vi "EOM.vi"(8 "error in (no error)":errorcluster, 9 "USE EOM?":bool, 10 "EOM_amplitude":dbl, 11 "Refnum in":refnum<k20>) -> (3 "EOM_out":dbl)   [LabVIEW 2018]
uses:
  <vilib>/Utility/error.llb/Error Cluster From Error Code.vi
  <vilib>/rvi/errors/niLvFpgaAdjustHostInterfaceError.vi
  <vilib>/rvi/interface/nirviReadWriteControl/nirviReadWriteControl.xnode
  Microspherefeedb_FPGATarget2_(FPGA)PIDXYZlase_Y-TtBVY85Jw.lvbitx
  NiFpgaLv.dll
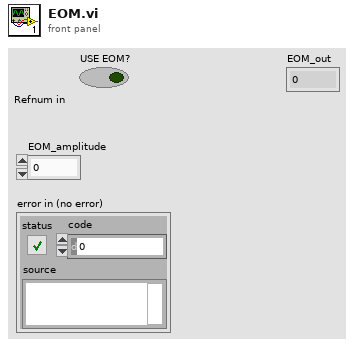
[diagram p1: front panel]
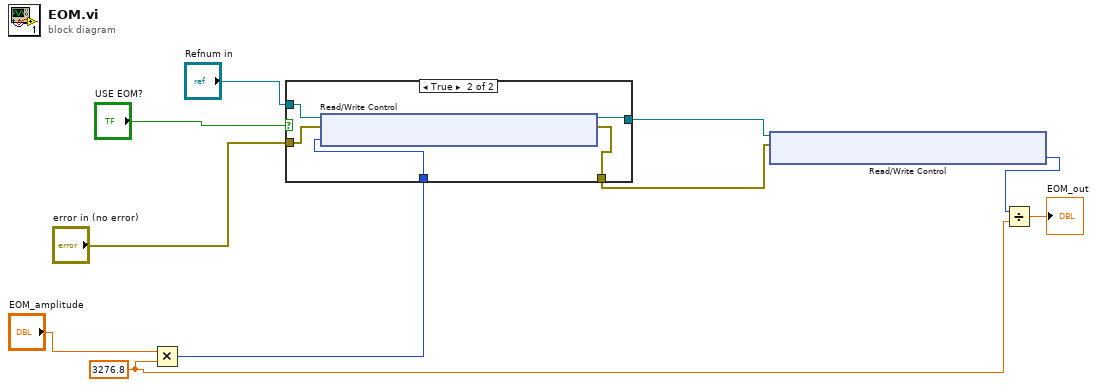
[diagram p0: block diagram]
diagram:
  w7 = 3276.8 ("y")
  n1 = Multiply(x="EOM_amplitude", y=w7) -> (x*y=w8:i16)
  n2 = case shown="True" "USE EOM?" {
    tunnel: "error in (no error)" -> [w12 w14]
    tunnel: w8 -> [_ w13]
    tunnel: [w12 w16] -> w1
    tunnel: "Refnum in" -> [w11 w17]
    tunnel: [w11 w15] -> w3
    frame False {
    }
    frame True {
      n3 = xnode "Read/Write Control"("FPGA VI Reference In"=w17, "error in"=w14, "EOM_amplitude"=w13) -> ("FPGA VI Reference Out"=w15:refnum<k20>, "error out"=w16:errorcluster)
    }
  }
  n4 = xnode "Read/Write Control"("FPGA VI Reference In"=w3, "error in"=w1) -> ("EOM_amplitude"=w2:i16)  [unwired: 2 out]
  n5 = Divide(x=w2, y=w7) -> (x/y=→"EOM_out":dbl)
